vi "Detection Logic to FPGA Modularized 2Player.vi"() -> ()   [LabVIEW 2026]
uses:
  <vilib>/rvi/Emulation/niFpgaGetClockAttributes.vi
  <vilib>/rvi/Emulation/niFpgaSctlEmulationGetInTimedLoop.vi
  <vilib>/rvi/Emulation/niFpgaEmulationReportErrorSimple.vi
  <vilib>/rvi/Emulation/niFpgaEmulationIsFPGAContextNoSignature.vi
  <vilib>/rvi/errors/niFpgaSetErrorForExecOnDevCompSimple.vi
  <vilib>/rvi/eio/common/nirviEmuReportErrorAndStop.vi
  <vilib>/rvi/DataTransferAndStorage/Container/Common/niFpgaContainerGetUniqueNameForEmu.vi
  <vilib>/rvi/FIFO/Fifo_Resource/nirvififoEmulationSetSize.vi
  <vilib>/rvi/FIFO/Fifo_Resource/nirviFifoEmulationQueueMgr.vi
  <instcachedir>/0/nirviFifoEmulationQueueMgr_E5CAEC123FF24DC58D834DCA3CDAA9B5.lvgen/nirviFifoEmulationQueueMgr_E5CAEC123FF24DC58D834DCA3CDAA9B5_000.vi
  <vilib>/Utility/error.llb/Clear Errors.vi
  <vilib>/rvi/FIFO/Fifo_Resource/nirvififoEmulationCreateLock.vi
  <vilib>/rvi/Emulation/niFpgaProcessEmulError.vi
  <vilib>/rvi/FIFO/Fifo_Resource/nirvififoEmulationObtainLock.vi
  <vilib>/rvi/FIFO/Fifo_Resource/nirvififoEmulationReleaseLock.vi
  <vilib>/rvi/occurrence/nirviWaitOnOccurrenceBase.vi
  <vilib>/rvi/errors/nirviReportUnexpectedCaseInternalError.vi
  <vilib>/rvi/errors/nirviReportUnexpectedCaseInternalError (U32).vi
  <instrlib>/_niInstr/Basic Elements/v1/FPGA/Private/Count Up U32.vi
  <vilib>/rvi/eio/common/nirviEmuTemplateMethod_errors.vi
  <vilib>/rvi/Emulation/niFpgaCriticalErrorInLSC.vi
  <extravilib>/ChannelInstances/Tag-bool/Instantiate.vi
  <extravilib>/ChannelInstances/Tag-u8/Instantiate.vi
  <vilib>/rvi/FIFO/Fifo_Resource/nirvififoEmulationDetermineInputValidOut.vi
  <vilib>/rvi/DataTransferAndStorage/Container/XNode/niFpgaContainer.xnode
  <vilib>/rvi/FIFO/Fifo_Resource/nirvififoEmulationRead.vi
  <vilib>/eio/EIONode/EIONode.xnode
  <vilib>/rvi/FIFO/Fifo_Resource/nirvififoEmulationWrite.vi
  <extravilib>/ChannelInstances/Tag-bool.lvlib
  <extravilib>/ChannelInstances/Tag-u8.lvlib
  <instrlib>/_niInstr/Basic Elements/v1/FPGA/niInstr Basic Elements v1 FPGA.lvlib
panel:
  in  "Frequency Array 2":fxp<+,32,0>[](array[numeric])=[1.100008375942707e-05, 1.165410503745079e-05, 1.3081356883049011e-05, 1.3859011232852936e-05, 1.7461366951465607e-05, 1.8499791622161865e-05, 2.1999934688210487e-05, 2.330821007490158e-05, 2.6162713766098022e-05, 2.7718255296349525e-05]
  in  "Frequency Array":fxp<+,32,0>[](array[numeric])=[1.100008375942707e-05, 1.165410503745079e-05, 1.3081356883049011e-05, 1.3859011232852936e-05, 1.7461366951465607e-05, 1.8499791622161865e-05, 2.1999934688210487e-05, 2.330821007490158e-05, 2.6162713766098022e-05, 2.7718255296349525e-05]
  in  "Blue-Green LEDs":u8[](array[numeric])=[0, 16, 24, 28, 30, 31]
  in  "Tone length2":u32=20000
  in  "Tone length1":u32=10000
  in  "Starting Lights":bool[](array[boolean])=[FALSE, FALSE, FALSE, FALSE, FALSE, FALSE, FALSE, FALSE, FALSE, FALSE, FALSE, FALSE, FALSE, FALSE, FALSE, FALSE, FALSE, FALSE, FALSE, FALSE, FALSE, FALSE, FALSE, FALSE, FALSE, FALSE, FALSE, FALSE, FALSE, FALSE, FALSE, FALSE, FALSE, FALSE, FALSE, FALSE, FALSE, FALSE, FALSE, FALSE, FALSE, FALSE, FALSE, FALSE, FALSE]
  out "Time Remaining":u32
  in  "Game Time, uS":u32 caption="Tick Count(uSec)"
  out "Score P2":u16
  out "Multiplier P2":u16
  out "Multiplier P1":u16
  out "Random Number":u8
  out "Score P1":u16
  in  "Speed Threshold, ticks":u64=3000
  in  "Debounce Threshold, ticks":u64=1000
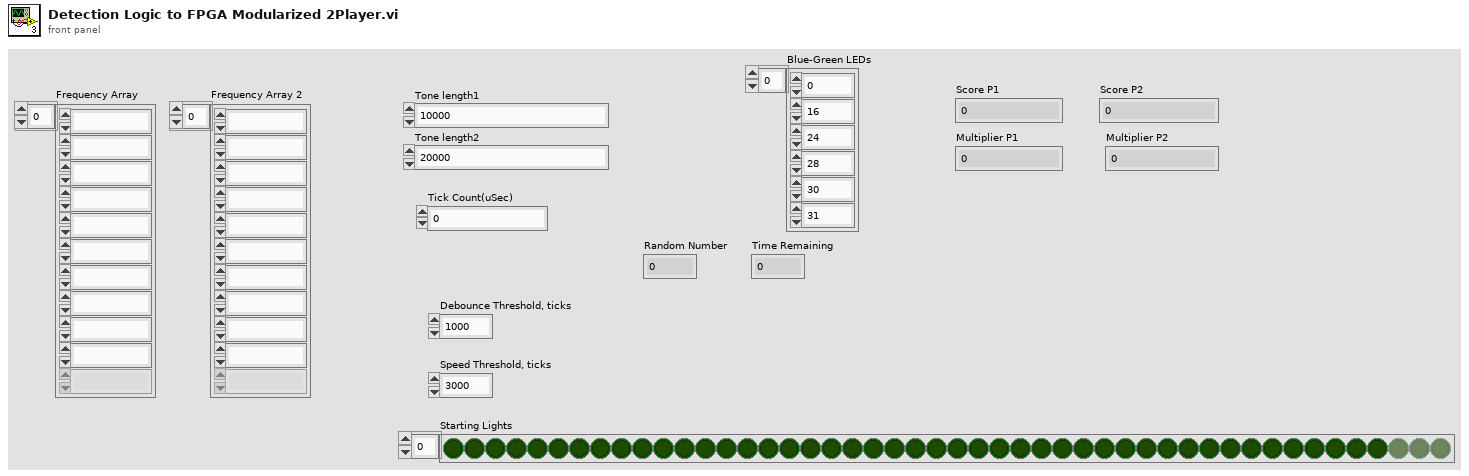
[diagram p1: front panel]
types:
  T1 = cluster{"Score":u16, "Multiplier":u16, "Last Press Tick":u64, u64[]}
  T2 = typedef "Tag-bool.lvlib/))Channel.ctl" = refnum<queue>
  T3 = cluster{"Score out":u16, "Multiplier out":u16, "Last Valid Press Tick out":u64, "Debounce Tick out":u64[]}
  T4 = typedef "Tag-u8.lvlib/))Channel.ctl" = refnum<queue>
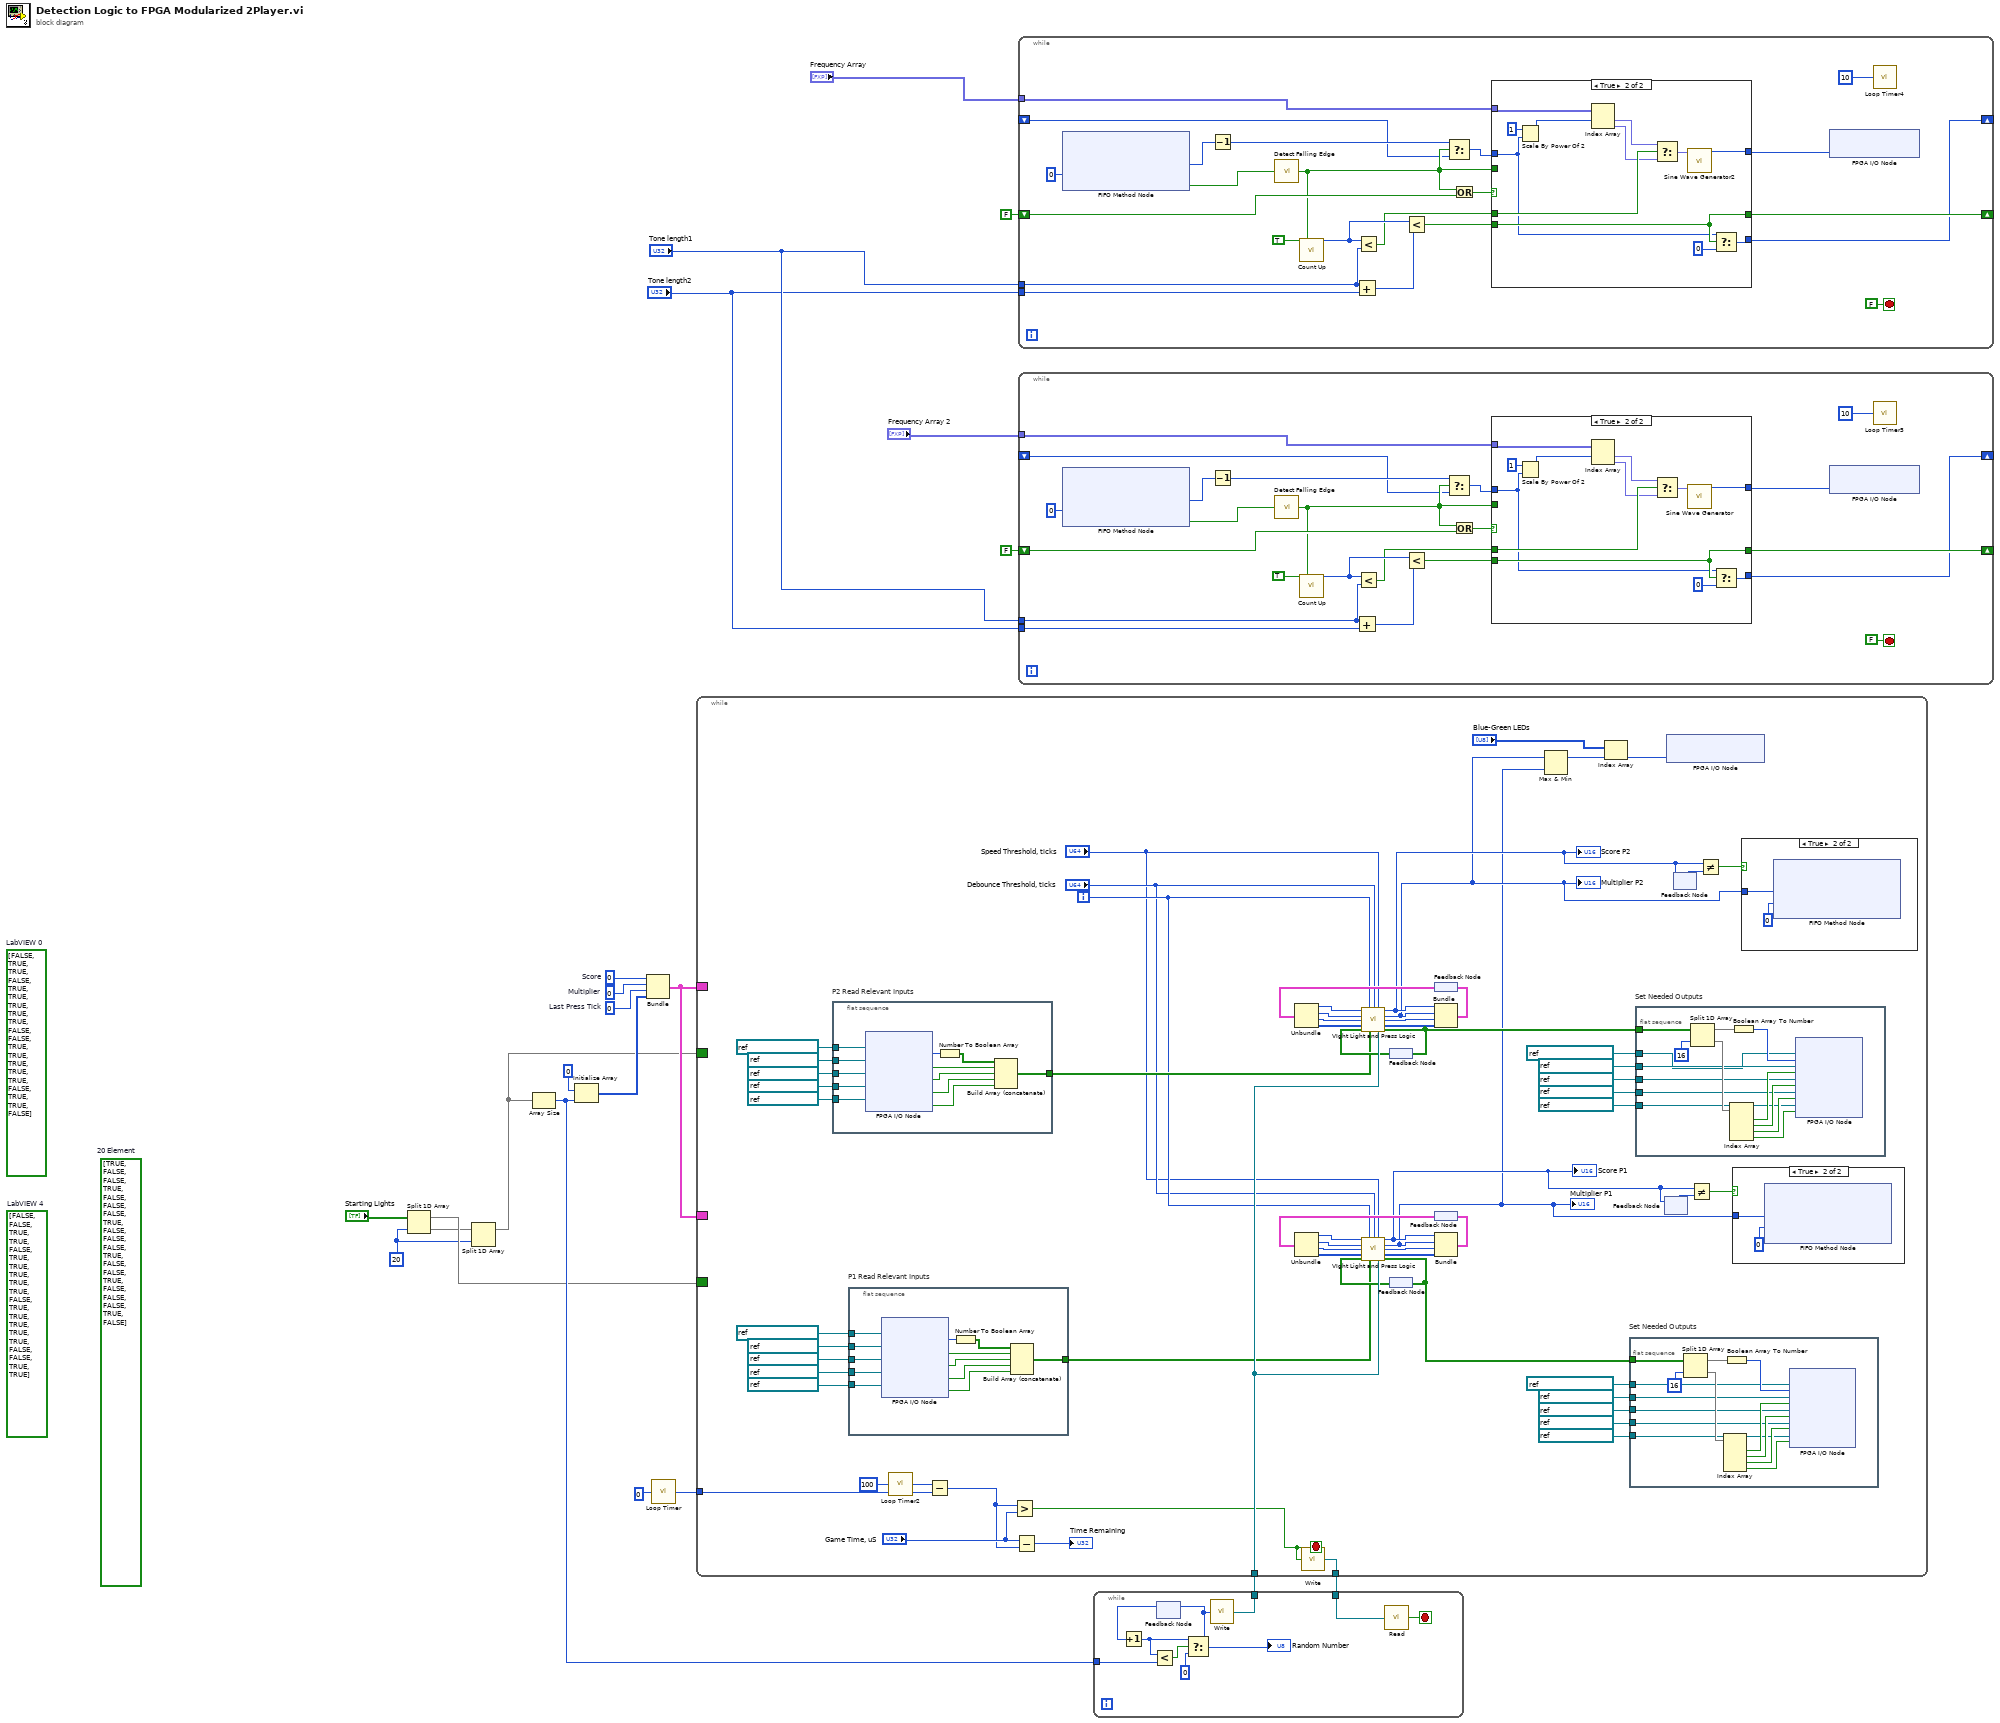
[diagram p0: block diagram]
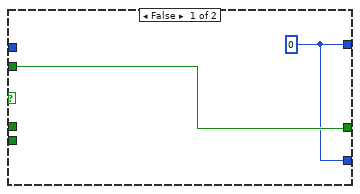
[diagram p2: hidden frame]
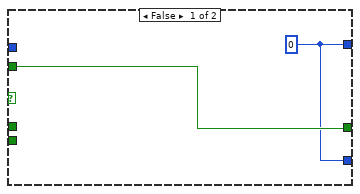
[diagram p3: hidden frame]
diagram:
  w8 = 20 ("index")
  (unwired) bool[] [FALSE, TRUE, TRUE, FALSE, TRUE, TRUE, TRUE, TRUE, TRUE, FALSE, FALSE, TRUE, TRUE, TRUE, TRUE, TRUE, FALSE, TRUE, TRUE, FALSE]  # LabVIEW 0
  (unwired) bool[] [FALSE, FALSE, TRUE, TRUE, FALSE, TRUE, TRUE, TRUE, TRUE, TRUE, FALSE, TRUE, TRUE, TRUE, TRUE, TRUE, FALSE, FALSE, TRUE, TRUE]  # LabVIEW 4
  w18 = u64 0  # Last Press Tick
  (unwired) bool[] [TRUE, FALSE, FALSE, TRUE, FALSE, FALSE, FALSE, TRUE, FALSE, FALSE, FALSE, TRUE, FALSE, FALSE, TRUE, FALSE, FALSE, FALSE, TRUE, FALSE]  # 20 Element
  w19 = u16 0  # Multiplier
  w20 = u16 0  # Score
  n1 = Split 1D Array(array="Starting Lights", index=w8) -> (first subarray=w10:bool[], second subarray=w9:bool[])
  n2 = Split 1D Array(array=w9, index=w8) -> (first subarray=w7:bool[])  [unwired: 1 out]
  n3 = Array Size(array=w7) -> (size(s)=w13:i32)
  n4 = Initialize Array(u64 0 ("Bonus Threshold"), w13) -> (w17:u64[])
  n5 = Bundle("Score"=w20, "Multiplier"=w19, "Last Press Tick"=w18, w17) -> (w16:T1)  [unwired: 1 in]
  n6 = call "Loop Timer"("Count(uSec)"=u32 0) -> ("Tick Count(uSec)"=w12:u32)
  n7 = while {
    tunnel: "Frequency Array" -> [w32]
    shift-right: [w36] -> _
    shift-left: FALSE ("edge detected") -> [w33]
    shift-right: [w30] -> _
    shift-left: _ -> [w27]
    tunnel: "Tone length2" -> [w24]
    tunnel: "Tone length1" -> [w23]
    stop <- FALSE stop-if-true
    n8 = xnode ("FIFO Method Node")("Timeout"=0) -> ("Element"=w41:u8, "Timed Out?"=w37:bool)  [unwired: 1 in, 1 out]
    n9 = Decrement(x=w41) -> (x-1=w29:u8)
    n10 = call <instrlib>:"Detect Falling Edge.vi"("signal"=w37) -> ("edge detected"=w28:bool)  [unwired: 14 in]
    n11 = call-poly <instrlib>:"Count Up.vi"("increment"=TRUE, "reset"=w28) -> ("count out"=w40:u32)  [unwired: 13 in]
    n12 = Add(x=w23, y=w24) -> (x+y=w25:u32)
    n13 = Less?(x=w40, y=w23) -> (x < y?=w38:bool)
    n14 = Less?(x=w40, y=w25) -> (x < y?=w34:bool)
    n15 = Select(t=w29, s=w28, f=w27) -> (s? t:f=w26:i16)
    n16 = Or(x=w28, y=w33) -> (x .or. y?=w35:bool)
    n17 = case shown="True" w35 {
      tunnel: w38 -> [_ w58]
      tunnel: [w45 w56] -> w31
      tunnel: w34 -> [_ w50]
      tunnel: [w46 w50] -> w36
      tunnel: w28 -> [w46 _]
      tunnel: w32 -> [_ w53]
      tunnel: [w45 w48] -> w30
      tunnel: w26 -> [_ w47]
      frame False {
        w45 = i16 0 ("SteroOut/AO1")
      }
      frame True {
        n18 = Scale By Power Of 2(n=i16 1, x=w47) -> (x*2^n=w55:i16)
        n19 = Index Array(array=w53, index #1=w55) -> (element #1=w52:fxp<+,32,0>, element #2=w51:fxp<+,32,0>)  [unwired: 1 in]
        n20 = Select(t=w52, s=w58, f=w51) -> (s? t:f=w57:fxp<+,32,0>)
        n21 = call "Sine Wave Generator2"("frequency (periods/tick)"=w57) -> ("sine out"=w56:i16)  [unwired: 14 in]
        n22 = Select(t=w47, s=w50, f=u8 0) -> (s? t:f=w48:i16)
      }
    }
    n23 = xnode "FPGA I/O Node"("SteroOut/AO0"=w31) -> ()  [unwired: 1 in, 1 out]
    n24 = call "Loop Timer4"("Count(uSec)"=u32 10 ("Count(Ticks)")) -> ()  [unwired: 1 out]
  }
  n25 = while {
    tunnel: "Frequency Array 2" -> [w68]
    shift-right: [w72] -> _
    shift-left: FALSE ("edge detected") -> [w69]
    shift-right: [w66] -> _
    shift-left: _ -> [w63]
    tunnel: "Tone length2" -> [w60]
    tunnel: "Tone length1" -> [w59]
    stop <- FALSE stop-if-true
    n26 = xnode ("FIFO Method Node")("Timeout"=0) -> ("Element"=w77:u8, "Timed Out?"=w73:bool)  [unwired: 1 in, 1 out]
    n27 = Decrement(x=w77) -> (x-1=w65:u8)
    n28 = call <instrlib>:"Detect Falling Edge.vi"("signal"=w73) -> ("edge detected"=w64:bool)  [unwired: 14 in]
    n29 = call-poly <instrlib>:"Count Up.vi"("increment"=TRUE, "reset"=w64) -> ("count out"=w76:u32)  [unwired: 13 in]
    n30 = Add(x=w59, y=w60) -> (x+y=w61:u32)
    n31 = Less?(x=w76, y=w59) -> (x < y?=w74:bool)
    n32 = Less?(x=w76, y=w61) -> (x < y?=w70:bool)
    n33 = Select(t=w65, s=w64, f=w63) -> (s? t:f=w62:i16)
    n34 = Or(x=w64, y=w69) -> (x .or. y?=w71:bool)
    n35 = case shown="True" w71 {
      tunnel: w74 -> [_ w94]
      tunnel: [w81 w92] -> w67
      tunnel: w70 -> [_ w86]
      tunnel: [w82 w86] -> w72
      tunnel: w64 -> [w82 _]
      tunnel: w68 -> [_ w89]
      tunnel: [w81 w84] -> w66
      tunnel: w62 -> [_ w83]
      frame False {
        w81 = i16 0 ("SteroOut/AO1")
      }
      frame True {
        n36 = Scale By Power Of 2(n=i16 1, x=w83) -> (x*2^n=w91:i16)
        n37 = Index Array(array=w89, index #1=w91) -> (element #1=w88:fxp<+,32,0>, element #2=w87:fxp<+,32,0>)  [unwired: 1 in]
        n38 = Select(t=w88, s=w94, f=w87) -> (s? t:f=w93:fxp<+,32,0>)
        n39 = call "Sine Wave Generator"("frequency (periods/tick)"=w93) -> ("sine out"=w92:i16)  [unwired: 14 in]
        n40 = Select(t=w83, s=w86, f=u8 0) -> (s? t:f=w84:i16)
      }
    }
    n41 = xnode "FPGA I/O Node"("SteroOut/AO1"=w67) -> ()  [unwired: 1 in, 1 out]
    n42 = call "Loop Timer3"("Count(uSec)"=u32 10 ("Count(Ticks)")) -> ()  [unwired: 1 out]
  }
  n43 = while {
    tunnel: [w158] -> w15
    border: w10 -> [_]
    tunnel: w21 -> [w159]
    border: w16 -> [_]
    border: w7 -> [_]
    border: w16 -> [_]
    tunnel: w12 -> [w109]
    i -> [w115]
    stop <- w110 stop-if-true
    n44 = flat-sequence "P2 Read Relevant Inputs" {
      tunnel: [w178] -> w127
      tunnel: refnum<k21> "Bank-03/DI7" ("FPGA I/O In") -> [w183]
      tunnel: refnum<k21> "Bank-03/DI6" ("FPGA I/O In") -> [w182]
      tunnel: refnum<k21> "Bank-03/DI5" ("FPGA I/O In") -> [w181]
      tunnel: refnum<k21> "Bank-03/DI4" ("FPGA I/O In") -> [w180]
      tunnel: refnum<k21> "Bank-02/DI15:0" ("FPGA I/O In") -> [w179]
      frame #0 {
        n45 = xnode "FPGA I/O Node"("FPGA I/O In"=w179, "FPGA I/O In"=w180, "FPGA I/O In"=w181, "FPGA I/O In"=w182, "FPGA I/O In"=w183) -> ("I/O Item"=w184:u16, "I/O Item"=w186:bool, "I/O Item"=w187:bool, "I/O Item"=w188:bool, "I/O Item"=w189:bool)  [unwired: 5 out]
        n46 = Number To Boolean Array(number=w184) -> (Boolean array=w185:bool[])
        n47 = Build Array (concatenate)(w185, w186, w187, w188, w189) -> (w178:bool[])
      }
    }
    n48 = flat-sequence "P1 Read Relevant Inputs" {
      tunnel: [w209] -> w147
      tunnel: refnum<k21> "Bank-03/DI3" ("FPGA I/O In") -> [w208]
      tunnel: refnum<k21> "Bank-03/DI2" ("FPGA I/O In") -> [w207]
      tunnel: refnum<k21> "Bank-03/DI1" ("FPGA I/O In") -> [w206]
      tunnel: refnum<k21> "Bank-03/DI0" ("FPGA I/O In") -> [w205]
      tunnel: refnum<k21> "Bank-01/DI15:0" ("FPGA I/O In") -> [w204]
      frame #0 {
        n49 = xnode "FPGA I/O Node"("FPGA I/O In"=w204, "FPGA I/O In"=w205, "FPGA I/O In"=w206, "FPGA I/O In"=w207, "FPGA I/O In"=w208) -> ("I/O Item"=w210:u16, "I/O Item"=w212:bool, "I/O Item"=w213:bool, "I/O Item"=w214:bool, "I/O Item"=w215:bool)  [unwired: 5 out]
        n50 = Number To Boolean Array(number=w210) -> (Boolean array=w211:bool[])
        n51 = Build Array (concatenate)(w211, w212, w213, w214, w215) -> (w209:bool[])
      }
    }
    n52 = call "Loop Timer2"("Count(uSec)"=u32 100) -> ("Tick Count(uSec)"=w111:u32)
    n53 = Subtract(x=w111, y=w109) -> (x-y=w107:u32)
    n54 = Greater?(x=w107, y="Game Time, uS") -> (0:w110:bool)
    n55 = Subtract(x="Game Time, uS", y=w107) -> (x-y=→"Time Remaining":u32)
    n56 = call <extravilib>:"Write.vi"("element"=w110) -> ("channel"=w158:T2)  [unwired: 1 out]
    n57 = feedback #1() -> (w138:bool[])
    n58 = feedback #2() -> (w157:bool[])
    n59 = feedback #3() -> (w142:T1)
    n60 = Unbundle(w142) -> ("Score"=w143:u16, "Multiplier"=w144:u16, "Last Press Tick"=w145:u64, w146:u64[])
    n61 = call "VIght Light and Press Logic.vi"("Score in"=w143, "Tick"=w115, "Debounce Threshold, ticks"="Debounce Threshold, ticks", "Speed Threshold, ticks"="Speed Threshold, ticks", "Multiplier in"=w144, "Last Valid Press Tick in"=w145, "Debounce Tick in"=w146, "Lit Buttons"=w138, "Pressed Buttons"=w127, "Random Number"=w159) -> ("Score out"=w103:u16, "Multiplier out"=w99:u16, "Last Valid Press Tick out"=w140:u64, "Debounce Tick out"=w139:u64[], "Buttons to Light"=w121:bool[])  [unwired: 1 in]
    "Score P2" <- w103
    "Multiplier P2" <- w99
    n62 = feedback-in #1(w121) -> ()
    n63 = Bundle("Score out"=w103, "Multiplier out"=w99, "Last Valid Press Tick out"=w140, "Debounce Tick out"=w139) -> (w141:T3)  [unwired: 1 in]
    n64 = feedback-in #3(w141) -> ()
    n65 = feedback #4() -> (w152:T1)
    n66 = Unbundle(w152) -> ("Score"=w151:u16, "Multiplier"=w150:u16, "Last Press Tick"=w149:u64, w148:u64[])
    n67 = call "VIght Light and Press Logic.vi"("Score in"=w151, "Tick"=w115, "Debounce Threshold, ticks"="Debounce Threshold, ticks", "Speed Threshold, ticks"="Speed Threshold, ticks", "Multiplier in"=w150, "Last Valid Press Tick in"=w149, "Debounce Tick in"=w148, "Lit Buttons"=w157, "Pressed Buttons"=w147, "Random Number"=w159) -> ("Score out"=w100:u16, "Multiplier out"=w98:u16, "Last Valid Press Tick out"=w154:u64, "Debounce Tick out"=w155:u64[], "Buttons to Light"=w156:bool[])  [unwired: 1 in]
    "Score P1" <- w100
    "Multiplier P1" <- w98
    n68 = feedback-in #2(w156) -> ()
    n69 = Bundle("Score out"=w100, "Multiplier out"=w98, "Last Valid Press Tick out"=w154, "Debounce Tick out"=w155) -> (w153:T3)  [unwired: 1 in]
    n70 = feedback-in #4(w153) -> ()
    n71 = Max & Min(x=w99, y=w98) -> (max(x,y)=w96:u16)  [unwired: 1 out]
    n72 = Index Array(array="Blue-Green LEDs", index=w96) -> (element=w95:u8)
    n73 = flat-sequence "Set Needed Outputs" {
      tunnel: w156 -> [w203]
      tunnel: refnum<k21> "Bank-03/DO3" ("FPGA I/O In") -> [w191]
      tunnel: refnum<k21> "Bank-03/DO2" ("FPGA I/O In") -> [w194]
      tunnel: refnum<k21> "Bank-03/DO1" ("FPGA I/O In") -> [w193]
      tunnel: refnum<k21> "Bank-03/DO0" ("FPGA I/O In") -> [w192]
      tunnel: refnum<k21> "Bank-01/DO15:0" ("FPGA I/O In") -> [w190]
      frame #0 {
        n74 = Split 1D Array(array=w203, index=16) -> (first subarray=w201:bool[], second subarray=w199:bool[])
        n75 = Index Array(array=w199) -> (element #1=w198:bool, element #2=w197:bool, element #3=w196:bool, element #4=w195:bool)  [unwired: 4 in]
        n76 = Boolean Array To Number(Boolean array=w201) -> (number=w202:u32)
        n77 = xnode "FPGA I/O Node"("I/O Item"=w202, "FPGA I/O In"=w190, "I/O Item"=w198, "FPGA I/O In"=w192, "I/O Item"=w197, "FPGA I/O In"=w193, "I/O Item"=w196, "FPGA I/O In"=w194, "I/O Item"=w195, "FPGA I/O In"=w191) -> ()  [unwired: 5 out]
      }
    }
    n78 = flat-sequence "Set Needed Outputs" {
      tunnel: w121 -> [w177]
      tunnel: refnum<k21> "Bank-03/DO7" ("FPGA I/O In") -> [w164]
      tunnel: refnum<k21> "Bank-03/DO6" ("FPGA I/O In") -> [w168]
      tunnel: refnum<k21> "Bank-03/DO5" ("FPGA I/O In") -> [w167]
      tunnel: refnum<k21> "Bank-03/DO4" ("FPGA I/O In") -> [w166]
      tunnel: refnum<k21> "Bank-02/DO15:0" ("FPGA I/O In") -> [w165]
      frame #0 {
        n79 = Split 1D Array(array=w177, index=16) -> (first subarray=w175:bool[], second subarray=w173:bool[])
        n80 = Index Array(array=w173) -> (element #1=w172:bool, element #2=w171:bool, element #3=w170:bool, element #4=w169:bool)  [unwired: 4 in]
        n81 = Boolean Array To Number(Boolean array=w175) -> (number=w176:u32)
        n82 = xnode "FPGA I/O Node"("I/O Item"=w176, "FPGA I/O In"=w165, "I/O Item"=w172, "FPGA I/O In"=w166, "I/O Item"=w171, "FPGA I/O In"=w167, "I/O Item"=w170, "FPGA I/O In"=w168, "I/O Item"=w169, "FPGA I/O In"=w164) -> ()  [unwired: 5 out]
      }
    }
    n83 = feedback #5() -> (w101:u16)  [unwired: 1 in]
    n84 = feedback-in #5(w100) -> ()
    n85 = xnode "FPGA I/O Node"("Bank-03/DO15:8"=w95) -> ()  [unwired: 1 in, 1 out]
    n86 = feedback #6() -> (w105:u16)  [unwired: 1 in]
    n87 = feedback-in #6(w103) -> ()
    n88 = Not Equal?(x=w100, y=w101) -> (x != y?=w102:bool)
    n89 = Not Equal?(x=w103, y=w105) -> (x != y?=w104:bool)
    n90 = case shown="True" w102 {
      tunnel: w98 -> [_ w160]
      frame False {
      }
      frame True {
        n91 = xnode ("FIFO Method Node")("Element"=w160, "Timeout"=0) -> ()  [unwired: 1 in, 2 out]
      }
    }
    n92 = case shown="True" w104 {
      tunnel: w99 -> [_ w162]
      frame False {
      }
      frame True {
        n93 = xnode ("FIFO Method Node")("Element"=w162, "Timeout"=0) -> ()  [unwired: 1 in, 2 out]
      }
    }
  }
  n94 = while {
    tunnel: w15 -> [w220]
    tunnel: w13 -> [w217]
    tunnel: [w216] -> w21
    stop <- w219 stop-if-true
    n95 = feedback #7() -> (w222:u8)  [unwired: 1 in]
    n96 = Increment(x=w222) -> (x+1=w218:u8)
    n97 = Less?(x=w218, y=w217) -> (x < y?=w223:bool)
    n98 = Select(t=w218, s=w223, f=u8 0) -> (s? t:f=w224:u8)
    "Random Number" <- w224
    n99 = feedback-in #7(w224) -> ()
    n100 = call <extravilib>:"Write.vi"("element"=w224) -> ("channel"=w216:T4)  [unwired: 1 out]
    n101 = call <extravilib>:"Read.vi"("channel"=w220) -> ("element"=w219:bool)  [unwired: 1 in, 1 out]
  }
